vi "TestDestroyIndex.vi"() -> (0 "Boolean":bool, 1 "Destroy Index":u32)   [LabVIEW 2009]
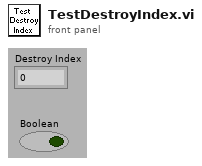
[diagram p1: front panel]
types:
  T1 = typedef "PickImage.ctl" = cluster{"Rawdata":T2, "Mask":T2, "Display":T2, "Coefficients (2D)":sgl[][], "Destroy Index":u32}
  T2 = typedef "IMAQ Image.ctl" = refnum<image>
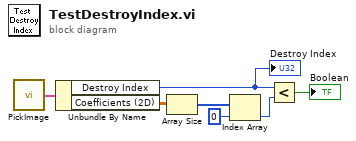
[diagram p0: block diagram]
diagram:
  n1 = call "PickImage.vi"() -> ("Image (output)"=w1:T1)  [unwired: 2 in]
  n2 = Unbundle By Name(w1) -> ("Destroy Index"=w2:u32, "Coefficients (2D)"=w3:sgl[][])
  "Destroy Index" <- w2
  n3 = Array Size(array=w3) -> (size(s)=w4:i32[])
  n4 = Index Array(array=w4, index=0) -> (element=w6:i32)
  n5 = Less?(x=w2, y=w6) -> (x < y?=→"Boolean":bool)
